vi "coupling_magnitude.vi"(4 "Reset":bool, 6 "High/low index":i32, 8 "Ref carrier amplitudes":T1 format="%#_3p", 9 "Sense amplitudes":T2 format="%#_3p", 10 "Carrier amplitudes":T5 format="%#_3p", 11 "Output options":T3) -> (3 "Magnitudes":dbl[](array[numeric]))   [LabVIEW 2026]
uses:
  processing/card_carrier_amplitudes.ctl
  gui/output_options.ctl
  gui/coupling_selector.ctl
  processing/card_high_carrier_amplitudes.ctl
  processing/carrier_amplitudes.ctl
panel:
  # "Coupling magnitude (scalar) across time"
  # "Sensor sample couplings"
  # "Current sense corresponding to \"Carrier amplitudes\""
  # "Reference amplitudes, only a single low rate measurement"
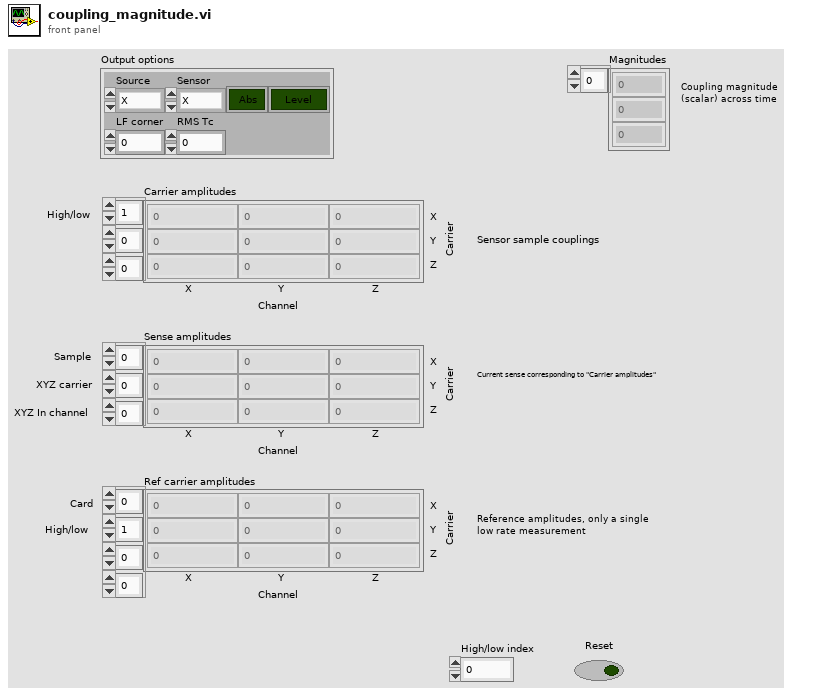
[diagram p1: front panel]
types:
  T1 = typedef "carrier_amplitudes.ctl" = cdb[][][][]
  T2 = typedef "card_high_carrier_amplitudes.ctl" = cdb[][][]
  T3 = typedef "output_options.ctl" = cluster{"Source":T4, "Sensor":T4, "Sense":bool, "Distance":bool, "LF corner":dbl, "RMS Tc":dbl}
  T4 = typedef "coupling_selector.ctl" = enum16{"X", "Y", "Z", "Vector"}
  T5 = typedef "card_carrier_amplitudes.ctl" = cdb[][][]
  T6 = typedef "coupling_matrix.ctl" = cdb[][]
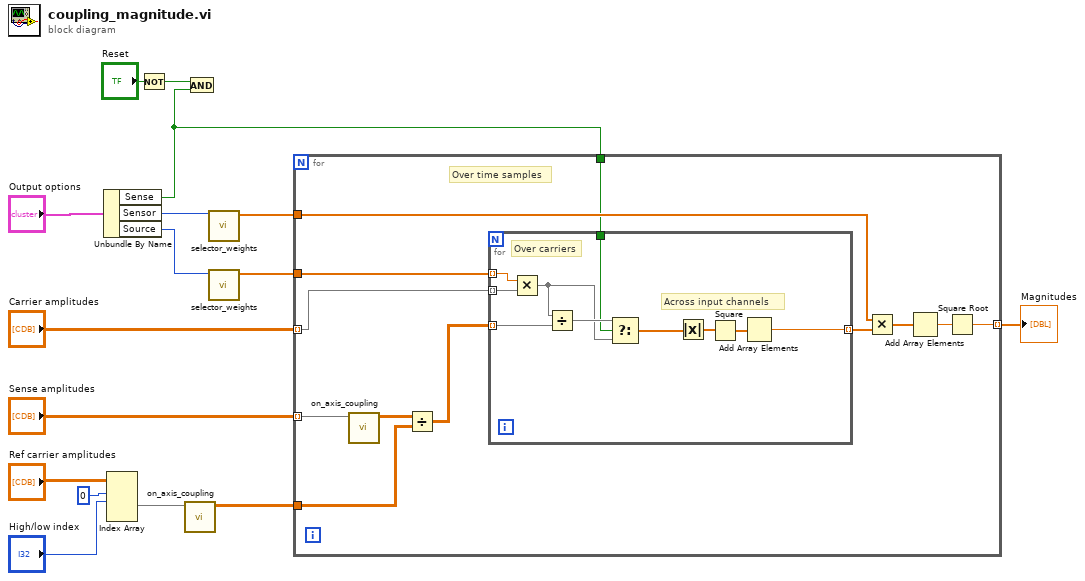
[diagram p0: block diagram]
diagram:
  n1 = Unbundle By Name("Output options") -> ("Sense"=w1:bool, "Sensor"=w11:T4, "Source"=w12:T4)
  n2 = Index Array(array="Ref carrier amplitudes", index (dim 0)=0 ("disabled index (vol)"), index (dim 1)="High/low index") -> (element=w3:cdb[][])  [unwired: 2 in]
  n3 = Not(x="Reset") -> (.not. x?=w8:bool)
  n4 = call "on_axis_coupling.vi"("Sense coupling"=w3) -> ("Sense amplitudes"=w2:T6)  [unwired: 10 in]
  n5 = And(x=w8, y=w1) -> ()  [unwired: 1 out]
  n6 = call "selector_weights.vi"("Selector"=w11) -> ("Weights"=w14:dbl[])  [unwired: 10 in]
  n7 = call "selector_weights.vi"("Selector"=w12) -> ("Weights"=w13:dbl[])  [unwired: 10 in]
  n8 = for {
    tunnel: "Carrier amplitudes" -> [w28] mode=indexing
    tunnel: "Sense amplitudes" -> [w19] mode=indexing
    tunnel: w13 -> [w25]
    tunnel: w14 -> [w26]
    tunnel: [w24] -> w9 mode=indexing
    tunnel: w1 -> [w21]
    tunnel: w2 -> [w18]
    # "Over time samples"
    n9 = call "on_axis_coupling.vi"("Sense coupling"=w19) -> ("Sense amplitudes"=w20:T6)  [unwired: 10 in]
    n10 = Divide(x=w20, y=w18) -> (x/y=w17:T6)
    n11 = for {
      tunnel: w28 -> [w33] mode=indexing
      tunnel: w17 -> [w38] mode=indexing
      tunnel: [w35] -> w27 mode=indexing
      tunnel: w25 -> [w34] mode=indexing
      tunnel: w21 -> [w30]
      # "Across input channels"
      # "Over carriers"
      n12 = Multiply(x=w34, y=w33) -> (x*y=w29:cdb[])
      n13 = Divide(x=w29, y=w38) -> (x/y=w32:cdb[])
      n14 = Select(t=w32, s=w30, f=w29) -> (s? t:f=w31:cdb[])
      n15 = Absolute Value(x=w31) -> (abs(x)=w37:dbl[])
      n16 = Square(x=w37) -> (x^2=w36:dbl[])
      n17 = Add Array Elements(numeric array=w36) -> (sum=w35:dbl)
    }
    n18 = Multiply(x=w26, y=w27) -> (x*y=w23:dbl[])
    n19 = Add Array Elements(numeric array=w23) -> (sum=w22:dbl)
    n20 = Square Root(x=w22) -> (sqrt(x)=w24:dbl)
  }
  "Magnitudes" <- w9
